vi "Inst.SPC.GetPublicEvents.vi"(8 "error in (no error)":errorcluster, 11 "Inst.SPC in":refnum<class "Inst.SPC.lvclass">) -> (0 "error out":errorcluster, 2 "Inst.SPC Public Events":T1, 3 "Inst.SPC out":refnum<class "Inst.SPC.lvclass">)   [LabVIEW 2019, in "Inst.SPC.lvclass"]
uses:
  Inst.SPC.lvclass
  Typedefs/PublicEvents--Cluster.ctl
  Typedefs/PublicEvents--Inst.SPC.MessageFromProcess.ctl
  <userlib>/LevyLab/Instrument Framework/SMOs/RemoteControl/Typedefs/Message--Cluster.ctl
  Inst.SPC.lvclass/Inst.SPC.ctl
  <userlib>/LevyLab/Instrument Framework/SMOs/RemoteControl/RemoteControl.lvclass
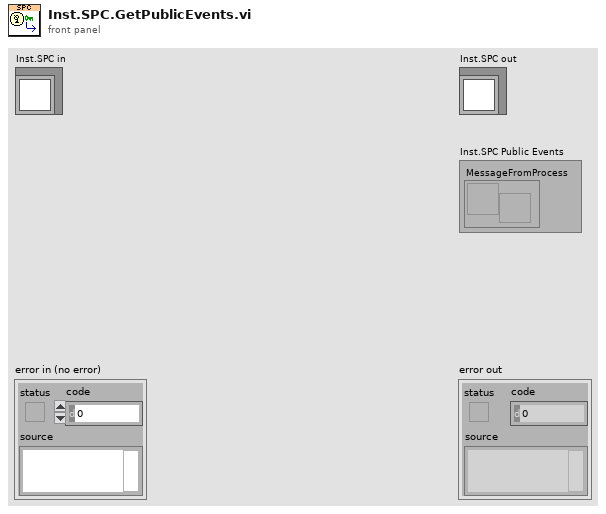
[diagram p1: front panel]
types:
  T1 = typedef "Inst.SPC.lvclass/PublicEvents--Cluster.ctl" = cluster{"MessageFromProcess":refnum<user-event>}
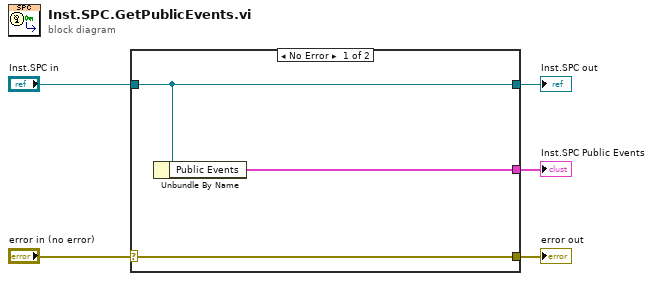
[diagram p0: block diagram]
diagram:
  n1 = case shown="No Error" "error in (no error)" {
    selector: "error in (no error)" -> [w8 w9]
    tunnel: [w8 w9] -> w4
    tunnel: [w7 w10] -> w2
    tunnel: "Inst.SPC in" -> [w7 w10]
    tunnel: [w6 _] -> w1
    frame No Error {
      n2 = Unbundle By Name(w7) -> ("Public Events"=w6:T1)
    }
    frame Error {
    }
  }
  "error out" <- w4
  "Inst.SPC out" <- w2
  "Inst.SPC Public Events" <- w1
